vi "Set XY Plot Properties on Variant.vi"(6 "Plot#":i32, 8 "error in (no error)":errorcluster, 10 "Plot":T1, 11 "variant in":variant) -> (0 "error out":errorcluster, 3 "variant out":variant)   [LabVIEW 2013, in "Workspace MultiY Graph.lvlib"]
uses:
  Workspace MultiY Graph.lvlib
  XY Plot Properties.ctl
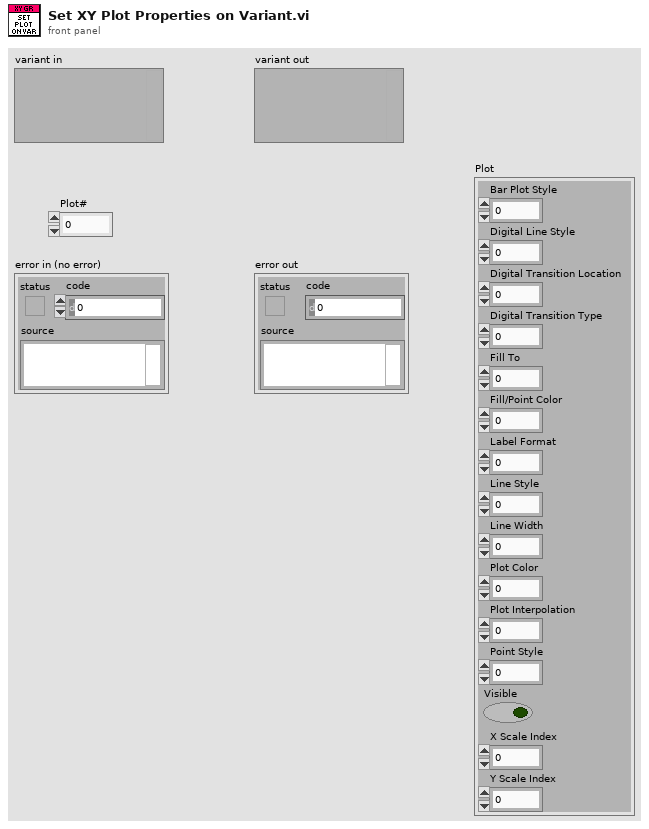
[diagram p1: front panel]
types:
  T1 = typedef "Workspace MultiY Graph.lvlib/XY Plot Properties.ctl" = cluster{"Bar Plot Style":u8, "Digital Line Style":u8, "Digital Transition Location":u8, "Digital Transition Type":u8, "Fill To":i16, "Fill/Point Color":u32, "Label Format":u8, "Line Style":u8, "Line Width":u8, "Plot Color":u32, "Plot Interpolation":u8, "Point Style":u8, "Visible":bool, "X Scale Index":u32, "Y Scale Index":u32}
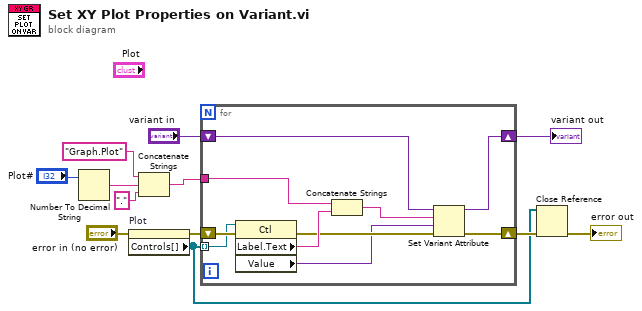
[diagram p0: block diagram]
diagram:
  n1 = Number To Decimal String(number="Plot#") -> (decimal integer string=w1:string)  [unwired: 1 in]
  n2 = property on="Plot" class="Clust (strict)"(error in="error in (no error)") -> (error out=w11:errorcluster, "Controls[]"=w7:refnum<vi>[])  [unwired: 1 in, 1 out]
  n3 = Concatenate Strings("Graph.Plot" ("name"), w1, "." ("string")) -> (w3:string)
  n4 = for {
    tunnel: w7 -> [w21] mode=indexing
    tunnel: w3 -> [w19]
    shift-right: [w20] -> w8
    shift-left: w11 -> [w22]
    shift-right: [w17] -> w9
    shift-left: "variant in" -> [w18]
    n5 = property on="Property Node" class="Ctl"(reference=w21, error in=w22) -> (error out=w15:errorcluster, "Label.Text"=w16:string, "Value"=w13:variant)  [unwired: 1 out]
    n6 = Concatenate Strings(w19, w16) -> (w14:string)
    n7 = Set Variant Attribute(Variant=w18, name=w14, value=w13, error in=w15) -> (Variant out=w17:variant, error out=w20:errorcluster)  [unwired: 1 out]
  }
  "variant out" <- w9
  n8 = Close Reference(reference=w7, error in (no error)=w8) -> (error out=→"error out":errorcluster)
